vi "Compressed Data Transfer Control (SubVI).vi"(0 "Bit-Depth In":u8, 1 "Minimum In":u8, 2 "BD-Min In Valid?":bool, 3 "Pixel Sync":bool, 4 "Data In":u64, 5 "Data In Valid?":bool, 6 "Record":bool, 8 "Image Width":u16, 10 "Image Height":u16) -> (12 "Packet Count":u32, 14 "Bit-Depth Out":u8, 15 "Minimum Out":u8, 16 "BD-Min Out Valid?":bool, 17 "Count Valid?":bool, 18 "Data Out":u64, 19 "Data Out Valid?":bool)   [LabVIEW 2015]
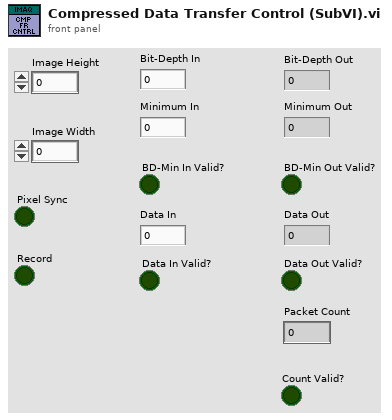
[diagram p1: front panel]
types:
  T1 = typedef "Pixel Bus.ctl" = cluster{"Pixel Valid":bool, "EOL":bool, "EOF":bool, "X":u16, "Y":u16}
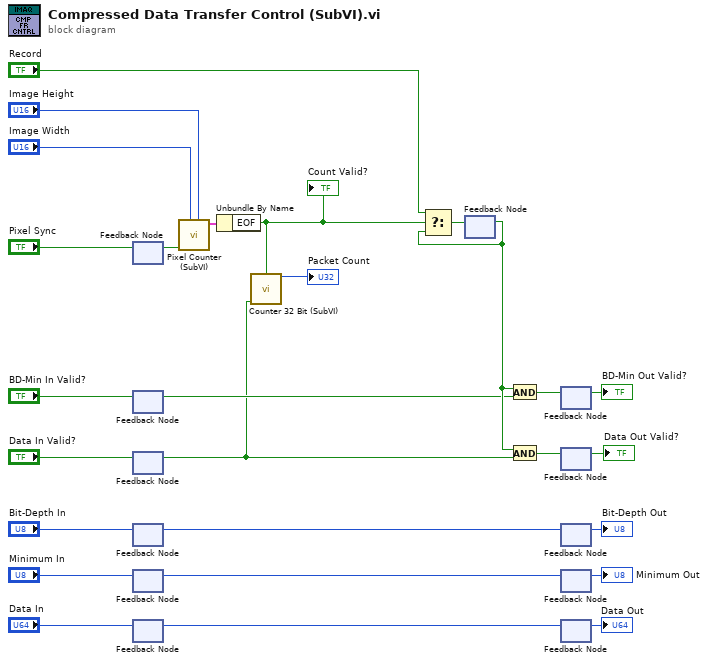
[diagram p0: block diagram]
diagram:
  n1 = feedback-in #1("Pixel Sync") -> ()
  n2 = feedback #1() -> (w6:bool)  [unwired: 1 in]
  n3 = feedback-in #2("BD-Min In Valid?") -> ()
  n4 = feedback #2() -> (w5:bool)  [unwired: 1 in]
  n5 = feedback-in #3("Data In Valid?") -> ()
  n6 = feedback #3() -> (w4:bool)  [unwired: 1 in]
  n7 = feedback-in #4("Bit-Depth In") -> ()
  n8 = feedback #4() -> (w3:u8)  [unwired: 1 in]
  n9 = feedback-in #5("Minimum In") -> ()
  n10 = feedback #5() -> (w2:u8)  [unwired: 1 in]
  n11 = feedback-in #6("Data In") -> ()
  n12 = feedback #6() -> (w1:u64)  [unwired: 1 in]
  n13 = call "Pixel Counter (SubVI).vi"("Image Height"="Image Height", "Image Width"="Image Width", "Pixel Valid"=w6) -> ("Pixel Bus"=w23:T1)  [unwired: 8 in]
  n14 = Unbundle By Name(w23) -> ("EOF"=w13:bool)
  "Count Valid?" <- w13
  n15 = call "Counter 32 Bit (SubVI).vi"("RESET"=w13, "Enable"=w4) -> ("Count"=→"Packet Count":u32)  [unwired: 11 in, 2 out]
  n16 = feedback #7() -> (w15:bool)  [unwired: 1 in]
  n17 = Select(t="Record", s=w13, f=w15) -> (s? t:f=w25:bool)
  n18 = feedback-in #7(w25) -> ()
  n19 = And(x=w15, y=w5) -> (x .and. y?=w27:bool)
  n20 = And(x=w15, y=w4) -> (x .and. y?=w16:bool)
  n21 = feedback-in #8(w27) -> ()
  n22 = feedback #8() -> (→"BD-Min Out Valid?":bool)  [unwired: 1 in]
  n23 = feedback #9() -> (→"Data Out Valid?":bool)  [unwired: 1 in]
  n24 = feedback-in #9(w16) -> ()
  n25 = feedback-in #10(w3) -> ()
  n26 = feedback #10() -> (→"Bit-Depth Out":u8)  [unwired: 1 in]
  n27 = feedback-in #11(w2) -> ()
  n28 = feedback #11() -> (→"Minimum Out":u8)  [unwired: 1 in]
  n29 = feedback-in #12(w1) -> ()
  n30 = feedback #12() -> (→"Data Out":u64)  [unwired: 1 in]
